vi "Check Disk Space.vi"() -> ()   [LabVIEW 2014]
panel:
  in  "stop":bool
  in  "Limit":dbl=20.0 format="%#_13g"
  out "Almost Full?":bool
  out "Free Percent":dbl
  out "free (bytes)":i64
  out "size (bytes)":i64
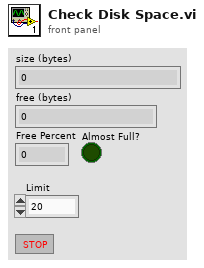
[diagram p1: front panel]
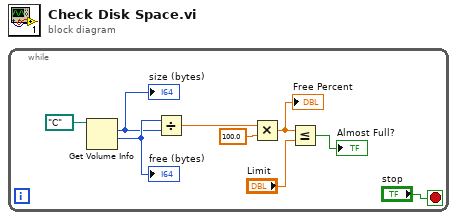
[diagram p0: block diagram]
diagram:
  n1 = while {
    stop <- "stop" stop-if-true
    n2 = Get Volume Info(11:path "C:/") -> (1:w8:i64, 2:w7:i64)  [unwired: 1 in, 4 out]
    "size (bytes)" <- w7
    "free (bytes)" <- w8
    n3 = Divide(x=w8, y=w7) -> (x/y=w6:dbl)
    n4 = Multiply(x=w6, y=100.0) -> (x*y=w4:dbl)
    "Free Percent" <- w4
    n5 = Less Or Equal?(x=w4, y="Limit") -> (x <= y?=→"Almost Full?":bool)
  }
